vi "Coerce To Limits.vi"(8 "error in (no error)":errorcluster, 9 "External Supply?":bool=TRUE, 10 "Power Supply In Use":T1, 11 "Channels to Coerce":T2[](array[typedef]) format="%.0x") -> (0 "error out":errorcluster, 3 "Values Coerced?":bool)   [LabVIEW 2018, in "NI PXI-4110 Programmable Power Supply Custom Device.lvlib"]
doc: "This VI takes in an array of channel references and then checks each channel to see if it's Voltage and Current properties match the currently selected hardware configuration. It returns a boolean value indicating whether any channels were changed."
uses:
  <vilib>/NI Veristand/Custom Device API/Custom Device Item Ref.ctl
  Power_Supply_In_Use.ctl
  4110_Global.vi
  <vilib>/NI Veristand/Custom Device API/Get Item Property (U16).vi
  <vilib>/NI Veristand/Custom Device API/Get Item Property (Double).vi
  <vilib>/NI Veristand/Custom Device API/Set Item Property (Double).vi
  NI PXI-4110 Programmable Power Supply Custom Device.lvlib
  <vilib>/NI VeriStand/Custom Device API/Custom Device API.lvlib
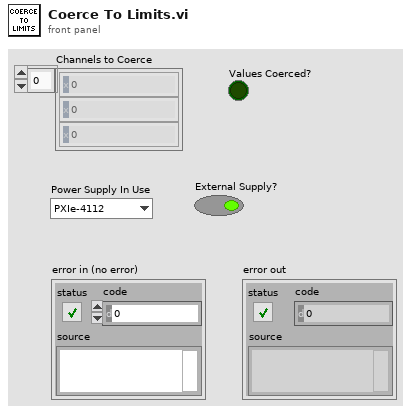
[diagram p1: front panel]
types:
  T1 = typedef "NI PXI-4110 Programmable Power Supply Custom Device.lvlib/Power_Supply_In_Use.ctl" = enum16{"PXIe-4112", "PXI-4110"}
  T2 = typedef "Custom Device API.lvlib/Custom Device Item Ref.ctl" = u64
  T3 = cluster{"V_min":dbl, "V_max":dbl, "I_min":dbl, "I_max":dbl}
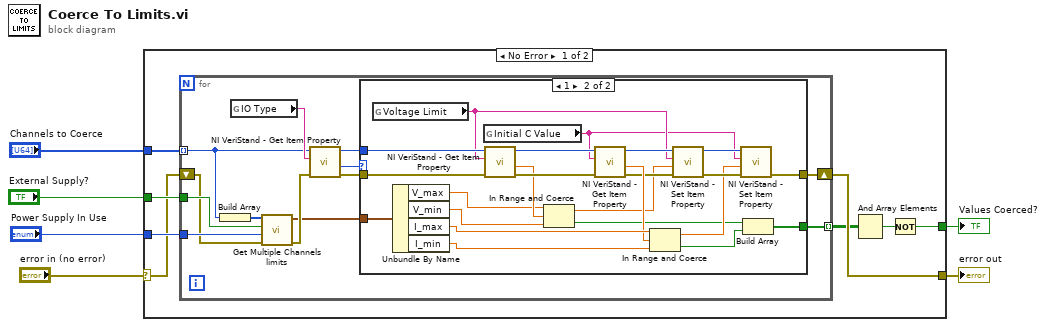
[diagram p0: block diagram]
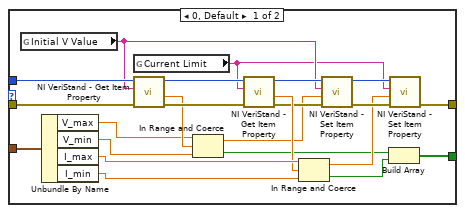
[diagram p2: hidden frame]
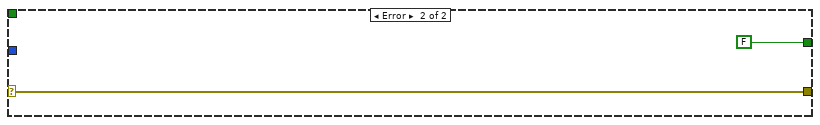
[diagram p3: hidden frame]
diagram:
  n1 = case shown="No Error" "error in (no error)" {
    selector: "error in (no error)" -> [w8 w75]
    tunnel: "Channels to Coerce" -> [w14 _]
    tunnel: [w11 w75] -> w4
    tunnel: "Power Supply In Use" -> [w13 _]
    tunnel: "External Supply?" -> [w12 _]
    tunnel: [w7 FALSE] -> w1
    frame No Error {
      n2 = for {
        tunnel: w14 -> [w23] mode=indexing
        tunnel: w13 -> [w22]
        tunnel: w12 -> [w20]
        shift-right: [w17] -> w11
        shift-left: w8 -> [w15]
        tunnel: [w16] -> w10 mode=indexing
        n3 = Build Array(w23) -> (w24:T2[])
        n4 = global read "4110_Global.vi" "IO Type"() -> (w27:string)
        n5 = call "Get Multiple Channels limits.vi"("error in (no error)"=w15, "Power Supply In Use"=w22, "External Supply?"=w20, "Channels"=w24) -> ("error out"=w21:errorcluster, "output cluster"=w18:T3)  [unwired: 6 in]
        n6 = call-poly <vilib>:"NI VeriStand - Get Item Property.vi"("error in (no error)"=w21, "Property Name"=w27, "Item Ref in"=w23) -> ("error out"=w19:errorcluster, "Value"=w26:u16, "Item Ref out"=w25:T2)  [unwired: 5 in, 1 out]
        n7 = case shown="1" w26 {
          tunnel: w25 -> [w50 w73]
          tunnel: w19 -> [w49 w72]
          tunnel: w18 -> [w45 w68]
          tunnel: [w31 w54] -> w17
          tunnel: [w30 w51] -> w16
          frame 0, Default {
            n8 = global read "4110_Global.vi" "Initial V Value"() -> (w36:string)
            n9 = Unbundle By Name(w45) -> ("V_max"=w44:dbl, "V_min"=w43:dbl, "I_max"=w42:dbl, "I_min"=w40:dbl)
            n10 = global read "4110_Global.vi" "Current Limit"() -> (w32:string)
            n11 = call-poly <vilib>:"NI VeriStand - Get Item Property.vi"("error in (no error)"=w49, "Property Name"=w36, "Item Ref in"=w50) -> ("error out"=w47:errorcluster, "Value"=w46:dbl, "Item Ref out"=w48:T2)  [unwired: 5 in, 1 out]
            n12 = In Range and Coerce(upper limit=w44, x=w46, lower limit=w43) -> (coerced(x)=w37:dbl, In Range?=w29:bool)
            n13 = call-poly <vilib>:"NI VeriStand - Get Item Property.vi"("error in (no error)"=w47, "Property Name"=w32, "Item Ref in"=w48) -> ("error out"=w38:errorcluster, "Value"=w41:dbl, "Item Ref out"=w39:T2)  [unwired: 5 in, 1 out]
            n14 = In Range and Coerce(upper limit=w42, x=w41, lower limit=w40) -> (coerced(x)=w33:dbl, In Range?=w28:bool)
            n15 = call-poly <vilib>:"NI VeriStand - Set Item Property.vi"("error in (no error)"=w38, "Value"=w37, "Property Name"=w36, "Item Ref in"=w39) -> ("error out"=w34:errorcluster, "Item Ref out"=w35:T2)  [unwired: 5 in, 1 out]
            n16 = Build Array(w29, w28) -> (w30:bool[])
            n17 = call-poly <vilib>:"NI VeriStand - Set Item Property.vi"("error in (no error)"=w34, "Value"=w33, "Property Name"=w32, "Item Ref in"=w35) -> ("error out"=w31:errorcluster)  [unwired: 5 in, 2 out]
          }
          frame 1 {
            n18 = global read "4110_Global.vi" "Voltage Limit"() -> (w59:string)
            n19 = Unbundle By Name(w68) -> ("V_max"=w67:dbl, "V_min"=w66:dbl, "I_max"=w65:dbl, "I_min"=w63:dbl)
            n20 = global read "4110_Global.vi" "Initial C Value"() -> (w55:string)
            n21 = call-poly <vilib>:"NI VeriStand - Get Item Property.vi"("error in (no error)"=w72, "Property Name"=w59, "Item Ref in"=w73) -> ("error out"=w70:errorcluster, "Value"=w69:dbl, "Item Ref out"=w71:T2)  [unwired: 5 in, 1 out]
            n22 = In Range and Coerce(upper limit=w67, x=w69, lower limit=w66) -> (coerced(x)=w60:dbl, In Range?=w53:bool)
            n23 = call-poly <vilib>:"NI VeriStand - Get Item Property.vi"("error in (no error)"=w70, "Property Name"=w55, "Item Ref in"=w71) -> ("error out"=w61:errorcluster, "Value"=w64:dbl, "Item Ref out"=w62:T2)  [unwired: 5 in, 1 out]
            n24 = In Range and Coerce(upper limit=w65, x=w64, lower limit=w63) -> (coerced(x)=w56:dbl, In Range?=w52:bool)
            n25 = call-poly <vilib>:"NI VeriStand - Set Item Property.vi"("error in (no error)"=w61, "Value"=w60, "Property Name"=w59, "Item Ref in"=w62) -> ("error out"=w57:errorcluster, "Item Ref out"=w58:T2)  [unwired: 5 in, 1 out]
            n26 = call-poly <vilib>:"NI VeriStand - Set Item Property.vi"("error in (no error)"=w57, "Value"=w56, "Property Name"=w55, "Item Ref in"=w58) -> ("error out"=w54:errorcluster)  [unwired: 5 in, 2 out]
            n27 = Build Array(w53, w52) -> (w51:bool[])
          }
        }
      }
      n28 = And Array Elements(Boolean array=w10) -> (logical AND=w9:bool)
      n29 = Not(x=w9) -> (.not. x?=w7:bool)
    }
    frame Error {
    }
  }
  "error out" <- w4
  "Values Coerced?" <- w1
